vi "Read Async Message.vi"(8 "error in (no error)":errorcluster, 11 "Completion Ack Msg in":refnum<class "Completion Notification Msg.lvclass">) -> (0 "error out":errorcluster, 2 "Async Methods Actor.lvlib:Async Message.lvclass":refnum<class "Async Message.lvclass">, 3 "Completion Ack Msg out":refnum<class "Completion Notification Msg.lvclass">)   [LabVIEW 2021, in "Async Methods Actor.lvlib" / "Completion Notification Msg.lvclass"]
uses:
  Completion Notification Msg.lvclass
  Async Message/Async Message.lvclass
  Completion Notification Msg.lvclass/Completion Notification Msg.ctl
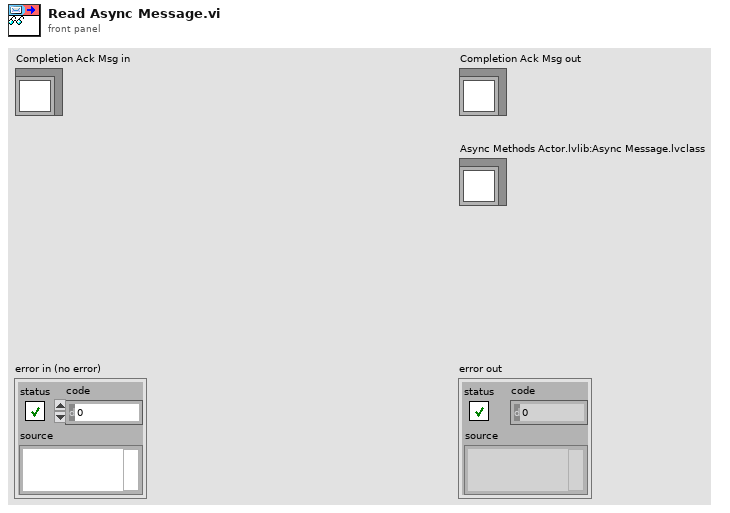
[diagram p1: front panel]
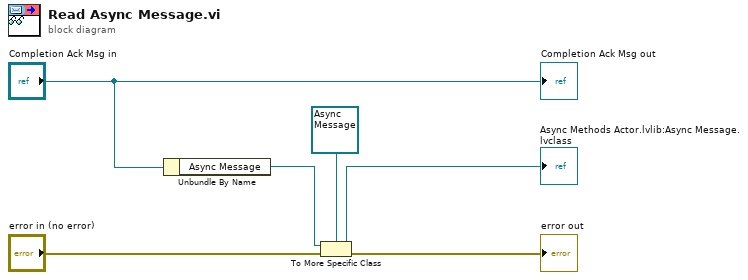
[diagram p0: block diagram]
diagram:
  n1 = Unbundle By Name("Completion Ack Msg in") -> ("Async Message"=w2:refnum<class "Message.lvclass">)
  n2 = To More Specific Class(target class=refnum<class "Async Message.lvclass"> refnum ("Async Methods Actor.lvlib:Async Message.lvclass"), reference=w2, error in="error in (no error)") -> (specific class reference=→"Async Methods Actor.lvlib:Async Message.lvclass":refnum<class "Async Message.lvclass">, error out=→"error out":errorcluster)
  "Completion Ack Msg out" <- "Completion Ack Msg in"
